vi "ventil zyklus.vi"() -> ()   [LabVIEW 2010]
panel:
  out "Position":i32
  out "Aktuelle Zeit":timestamp
  out "Durchlauf Nr.":i32
  in  "?":bool
  in  "Positionen (1-6)":i32[](array[numeric])=[1, 3, 5, 2]
  out "Anzahl der Zustände":i32
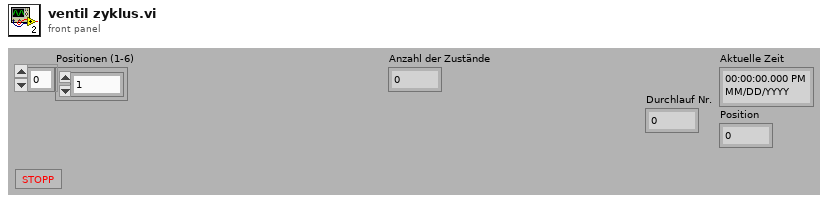
[diagram p1: front panel]
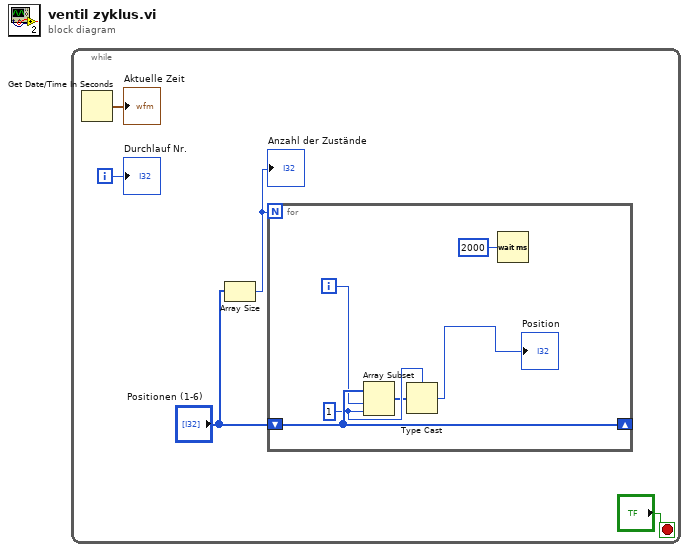
[diagram p0: block diagram]
diagram:
  n1 = while {
    i -> [w2]
    stop <- "?" stop-if-true
    n2 = Get Date/Time In Seconds() -> (seconds since 1Jan1904=→"Aktuelle Zeit":timestamp)
    n3 = Array Size(array="Positionen (1-6)") -> (size(s)=w4:i32)
    "Anzahl der Zustände" <- w4
    n4 = for {
      N: w4 -> [_]
      shift-right: [w11] -> _
      shift-left: "Positionen (1-6)" -> [w11]
      i -> [w7]
      w10 = 1 ("Länge")
      n5 = Array Subset(array=w11, index=w7, length=w10) -> (w9:i32[])
      n6 = Type Cast(type=w10, x=w9) -> (*(type *) &x=→"Position":i32)
      n7 = Wait (ms)(milliseconds to wait=u32 2000 ("Zu wartende ms")) -> ()  [unwired: 1 out]
    }
    "Durchlauf Nr." <- w2
  }
